vi "AssignStatus.vi"(5 "LoopCount":dbl, 6 "Time":u32, 7 "Init Val":dbl, 8 "error in (no error)":errorcluster, 9 "ROSCO Params":T3, 10 "?":T1={"iSTATUS"=0, "TIME"=1, "DT"=2, "BL_PITCH_1"=3, "VS_MECHGENPWR"=13, "GEN_SPEED"=19, "ROT_SPEED"=20, "GENTQMEAS"=22, "Y_M"=23, "HORWINDV"=26, "ROOTMOOP1"=29, "ROOTMOOP2"=30, "BL_PITCH_2"=32, "BL_PITCH_3"=33, "ROOTMOOP3"=31, "INFILE_SIZE"=49, "FA_ACC"=52, "NUM_BLADES"=60, " OUT BL_PITCH"=44, "OUT_ TORQUE"=46, "OUTFILE_SIZE "=50, "AVCMSG_SIZE"=48, "AERODYN TQ"=89, "VS_GENPWR"=13}, 11 "SwapIn":T2) -> (0 "error out":errorcluster, 1 "ROSCO Params 2":T3, 2 "?":T1={"iSTATUS"=0, "TIME"=1, "DT"=2, "BL_PITCH_1"=3, "VS_MECHGENPWR"=13, "GEN_SPEED"=19, "ROT_SPEED"=20, "GENTQMEAS"=22, "Y_M"=23, "HORWINDV"=26, "ROOTMOOP1"=29, "ROOTMOOP2"=30, "BL_PITCH_2"=32, "BL_PITCH_3"=33, "ROOTMOOP3"=31, "INFILE_SIZE"=49, "FA_ACC"=52, "NUM_BLADES"=60, " OUT BL_PITCH"=44, "OUT_ TORQUE"=46, "OUTFILE_SIZE "=49, "AVCMSG_SIZE"=49, "AERODYN TQ"=46, "VS_GENPWR"=13}, 3 "SwapIn":T2, 4 "Count+1":dbl)   [LabVIEW 2018]
uses:
  Clusters/SwapIn.ctl
  Clusters/RoscoParams.ctl
  Clusters/SwapIndexes.ctl
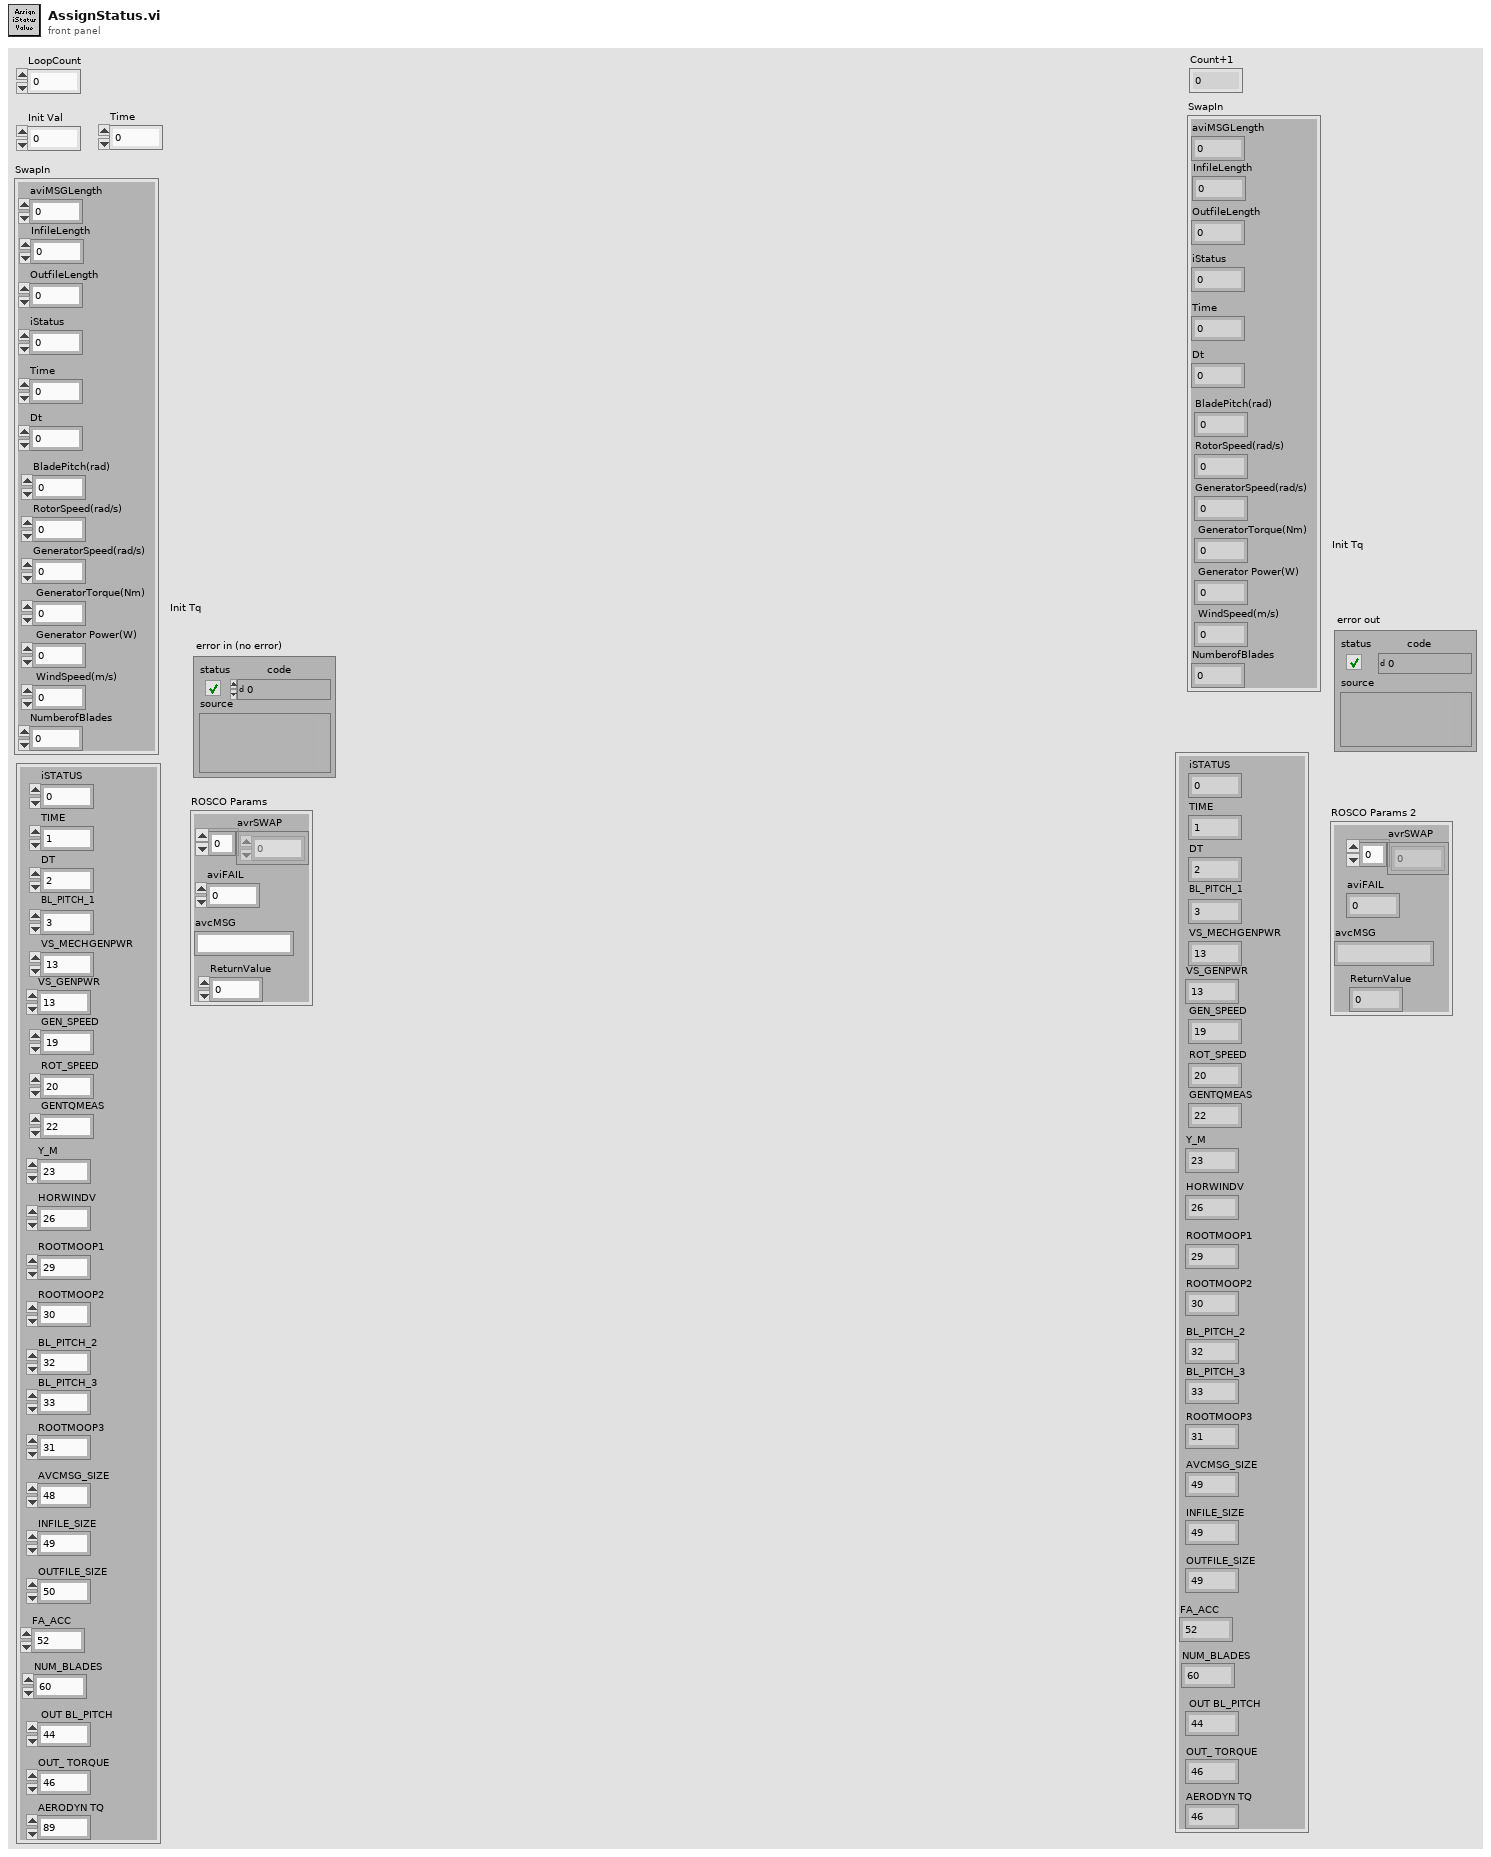
[diagram p1: front panel]
types:
  T1 = typedef "SwapIndexes.ctl" = cluster{"iSTATUS":i32, "TIME":i32, "DT":i32, "BL_PITCH_1":i32, "VS_MECHGENPWR":i32, "GEN_SPEED":i32, "ROT_SPEED":i32, "GENTQMEAS":i32, "Y_M":i32, "HORWINDV":i32, "ROOTMOOP1":i32, "ROOTMOOP2":i32, "BL_PITCH_2":i32, "BL_PITCH_3":i32, "ROOTMOOP3":i32, "INFILE_SIZE":i32, "FA_ACC":i32, "NUM_BLADES":i32, " OUT BL_PITCH":i32, "OUT_ TORQUE":i32, "OUTFILE_SIZE ":i32, "AVCMSG_SIZE":i32, "AERODYN TQ":i32, "VS_GENPWR":i32}
  T2 = typedef "SwapIn.ctl" = cluster{"BladePitch(rad)":sgl, "RotorSpeed(rad/s)":sgl, "GeneratorSpeed(rad/s)":sgl, " GeneratorTorque(Nm)":sgl, " Generator Power(W) ":sgl, " WindSpeed(m/s)":sgl, "aviMSGLength":sgl, "InfileLength":sgl, "OutfileLength":sgl, "iStatus":sgl, "Time":sgl, "Dt":sgl, "NumberofBlades":sgl}
  T3 = typedef "RoscoParams.ctl" = cluster{"avrSWAP":sgl[], "aviFAIL":i32, "avcMSG":string, "ReturnValue":i32}
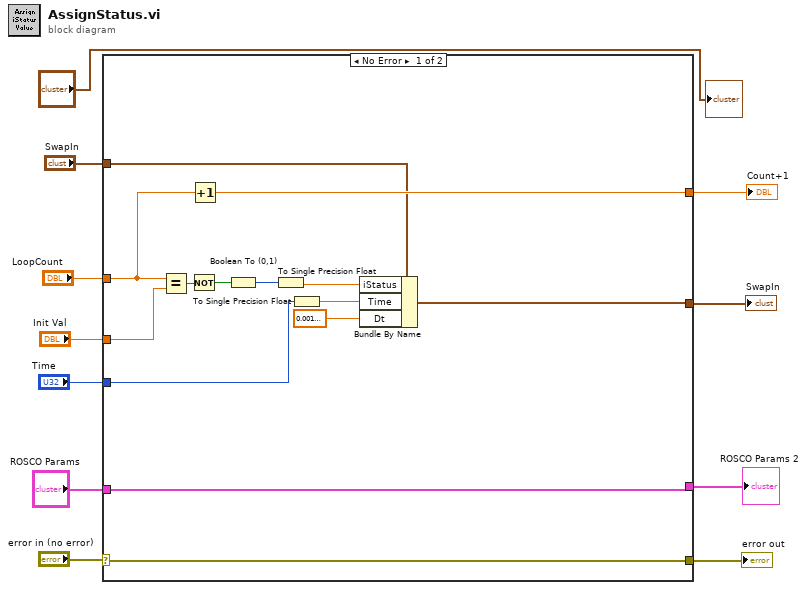
[diagram p0: block diagram]
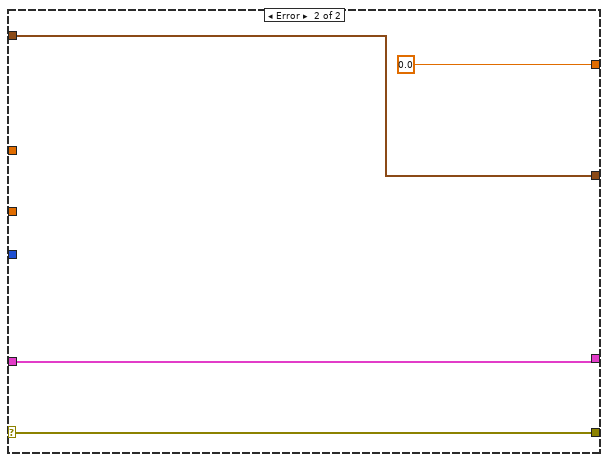
[diagram p2: hidden frame]
diagram:
  n1 = case shown="No Error" "error in (no error)" {
    selector: "error in (no error)" -> [w18 w29]
    tunnel: [w25 w27] -> w11
    tunnel: [w21 0.0] -> w10
    tunnel: "LoopCount" -> [w13 _]
    tunnel: "Init Val" -> [w20 _]
    tunnel: [w18 w29] -> w6
    tunnel: [w17 w26] -> w4
    tunnel: "ROSCO Params" -> [w17 w26]
    tunnel: "SwapIn" -> [w16 w27]
    tunnel: "Time" -> [w12 _]
    frame No Error {
      n2 = Equal?(x=w13, y=w20) -> (x = y?=w19:bool)
      n3 = Not(x=w19) -> (.not. x?=w23:bool)
      n4 = Increment(x=w13) -> (x+1=w21:dbl)
      n5 = Boolean To (0,1)(Boolean=w23) -> (0, 1=w22:i16)
      n6 = To Single Precision Float(number=w22) -> (single precision float=w24:sgl)
      n7 = To Single Precision Float(number=w12) -> (single precision float=w15:sgl)
      n8 = Bundle By Name(cluster=w16, "iStatus"=w24, "Time"=w15, "Dt"=sgl 0.001) -> (w25:T2)
    }
    frame Error {
    }
  }
  "SwapIn" <- w11
  "Count+1" <- w10
  "error out" <- w6
  "ROSCO Params 2" <- w4
  "?" <- "?"
